vi "SHA-1_hash chunk_U32.vi"(0 "h0":u32 format="%.0x", 1 "Chunk":u32[](array[numeric]), 5 "h1":u32, 7 "h2":u32, 9 "h3":u32, 11 "h4":u32, 12 "error in (no error)":errorcluster) -> (4 "a":u32, 6 "b":u32, 8 "c":u32, 10 "d":u32, 14 "error out":errorcluster, 15 "e":u32)   [LabVIEW 2012, in "Encryption.lvlib"]
uses:
  Encryption.lvlib
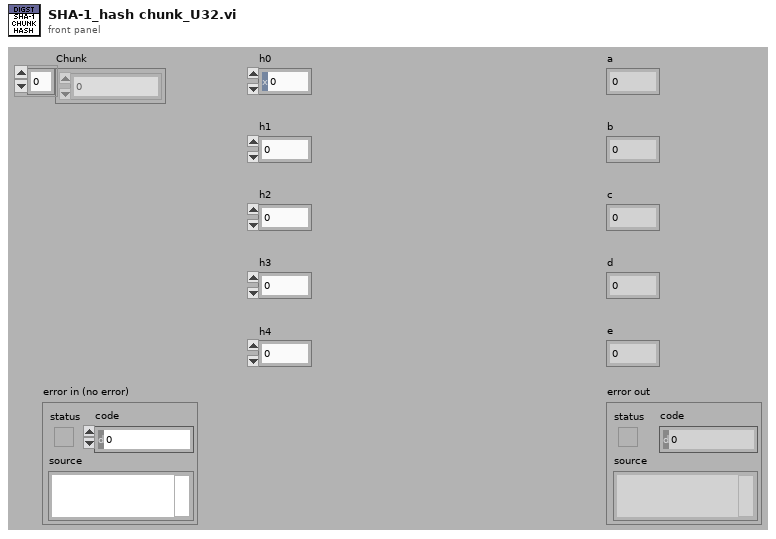
[diagram p1: front panel]
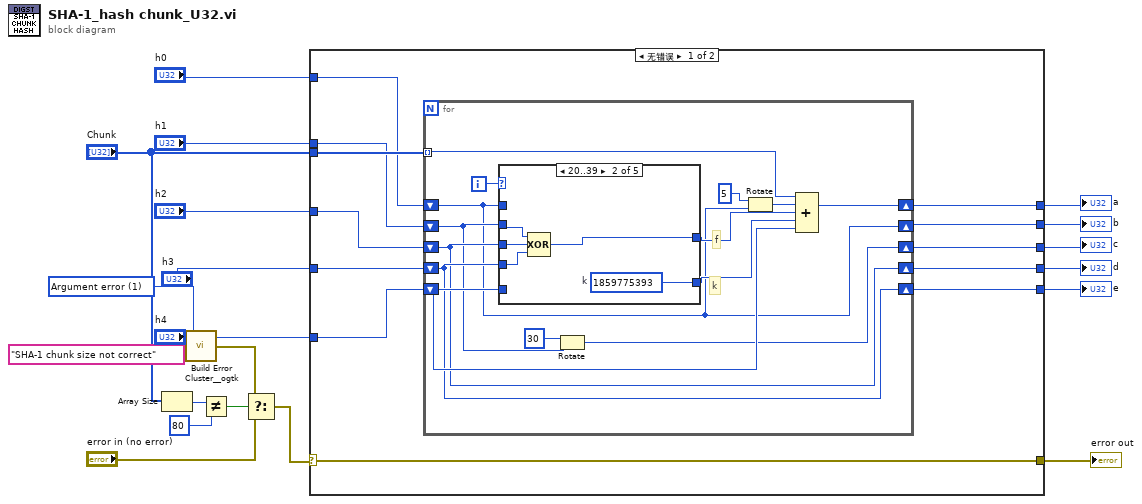
[diagram p0: block diagram]
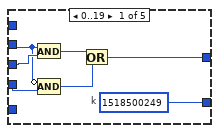
[diagram p2: hidden frame]
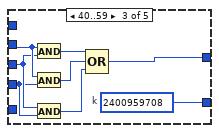
[diagram p3: hidden frame]
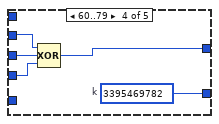
[diagram p4: hidden frame]
diagram:
  w11 = 1 items=["No error", "Argument error", "Memory is full", "Out of zone", "End of file", "File already open", "Generic file I/O error", "File not found", "File permission error", "Disk is full", "Duplicate path", "Too many files open", "System feature not enabled", "Resource file not found", "Cannot add resource", "Resource not found", "Image not found", "Image memory error", "Pen does not exist", "Config type invalid", "Config token not found", "Config parse error", "Config memory error", "Bad external code format", "Bad external code offset", "External code not present", "Null window", "Destroy window error", "Null menu", "Print aborted", "Bad print record", "Print driver error", "Windows error during printing", "Memory error during printing", "Print dialog error", "Generic print error", "Invalid device refnum", "Device not found", "Device parameter error", "Device unit error", "Cannot open device", "Device call aborted", "Generic error", "Cancelled by user", "Object ID too low", "Object ID too high", "Object not in heap", "Unknown heap", "Unknown object (invalid DefProc)", "Unknown object (DefProc not in table)", "Message out of range", "Invalid (null) method", "Unknown message", "Manager call not supported", "Bad address", "Network operation in progress", "Network operation timed out", "Connection is busy", "Network attribute not supported", "Network error", "Address in use", "System out of memory", "Connection aborted", "Connection refused", "Not connected", "Already connected", "Connection closed", "Initialization error (interapplication manager)", "Bad occurrence", "Wait on unbound occurrence handler", "Occurrence queue overflow", "Datalog type conflict", "Unused", "Unrecognized type (interapplication manager)", "Memory corrupt", "Failed to make temporary DLL", "Old CIN version", "Drag socket not found", "Failed to load drop-object", "Failed to register OLE object", "Failed to release OLE object", "Format specifier type mismatch", "Unknown format specifier", "Too few format specifiers", "Too many format specifiers", "Scan failed", "Newer CIN version", "Error converting to variant", "Runtime menu error", "Password tampered", "Variant attribute not found", "Incompatible variant data type", "Event data is not available", "Event Store is not present", "Occurrence is not found", "Event Queue is not created", "Event info is not available", "Refnum passed is NULL", "Error retrieving Class GUID", "Error retrieving CoClass GUID", "Error retrieving TypeLib GUID.", "Bad built application magic bytes.", "Specific driver is different from the specific driver associated with the Logical Name.", "There is no session opened to the class driver.", "Max Error", "MAX - Error with config objects", "MAX - Error loading configuration", "MAX - Group not supported"]
  n1 = Array Size(array="Chunk") -> (size(s)=w19:i32)
  n2 = call <userlib>:"Build Error Cluster__ogtk.vi"("String to Prepend to source (\"\")"="SHA-1 chunk size not correct" ("String to Prepend to source (\"\")"), "code"=w11) -> ("error out"=w13:errorcluster)
  n3 = Not Equal?(x=w19, y=80) -> (x != y?=w17:bool)
  n4 = Select(t=w13, s=w17, f="error in (no error)") -> (s? t:f=w15:errorcluster)
  n5 = case shown="无错误" w15 {
    selector: w15 -> [w31 w72]
    tunnel: "Chunk" -> [w32 _]
    tunnel: [w31 w72] -> w14
    tunnel: [w30 _] -> w10
    tunnel: [w29 _] -> w9
    tunnel: [w28 _] -> w8
    tunnel: [w27 _] -> w7
    tunnel: [w26 _] -> w6
    tunnel: "h0" -> [w25 _]
    tunnel: "h1" -> [w24 _]
    tunnel: "h2" -> [w23 _]
    tunnel: "h3" -> [w22 _]
    tunnel: "h4" -> [w21 _]
    frame No Error {
      n6 = for {
        tunnel: w32 -> [w33] mode=indexing
        shift-right: [w34] -> w29
        shift-left: w25 -> [w35]
        shift-right: [w35] -> w28
        shift-left: w24 -> [w37]
        shift-right: [w36] -> w27
        shift-left: w23 -> [w39]
        shift-right: [w39] -> w26
        shift-left: w22 -> [w40]
        shift-right: [w40] -> w30
        shift-left: w21 -> [w41]
        i -> [w46]
        # "k"
        # "f"
        n7 = case shown="20..39" w46 {
          tunnel: w35 -> [_ _ _ _ _]
          tunnel: w37 -> [w52 w55 w66 w68 _]
          tunnel: w39 -> [w53 w54 w61 w67 _]
          tunnel: w40 -> [w51 w58 w60 w71 _]
          tunnel: w41 -> [_ _ _ _ _]
          tunnel: [w48 w56 w63 w69 _] -> w43
          tunnel: [w47 w57 w62 w70 _] -> w42
          frame 0..19 {
            w47 = u32 1518500249  # k
            n8 = And(x=w52, y=w53) -> (x .and. y?=w49:u32)
            n9 = Compound Arithmetic op=AND(invert w52, w51) -> (w50:u32)
            n10 = Or(x=w49, y=w50) -> (x .or. y?=w48:u32)
          }
          frame 20..39 {
            w57 = u32 1859775393  # k
            n11 = Compound Arithmetic op=XOR(w55, w54, w58) -> (w56:u32)
          }
          frame 40..59 {
            w62 = u32 2400959708  # k
            n12 = And(x=w66, y=w61) -> (x .and. y?=w64:u32)
            n13 = And(x=w66, y=w60) -> (x .and. y?=w65:u32)
            n14 = And(x=w61, y=w60) -> (x .and. y?=w59:u32)
            n15 = Compound Arithmetic op=OR(w64, w65, w59) -> (w63:u32)
          }
          frame 60..79 {
            w70 = u32 3395469782  # k
            n16 = Compound Arithmetic op=XOR(w68, w67, w71) -> (w69:u32)
          }
          frame Default {
          }
        }
        n17 = Rotate(1:w37, 2:i8 30 ("y")) -> (0:w36:u32)
        n18 = Rotate(1:w35, 2:i8 5 ("y")) -> (0:w44:u32)
        n19 = Compound Arithmetic op=ADD(w33, w44, w43, w42, w41) -> (w34:u32)
      }
    }
    frame Error {
    }
  }
  "error out" <- w14
  "d" <- w6
  "c" <- w7
  "b" <- w8
  "a" <- w9
  "e" <- w10
